vi "DAQ Channels Names.vi"() -> (6 "DAQ channel names (string)":string[](array[string]))   [LabVIEW 2017, in "SignalConverson.lvlib"]
uses:
  SignalConverson.lvlib
  DAQChannelRawData.ctl
panel:
  in  "ChannelNameArray":T1
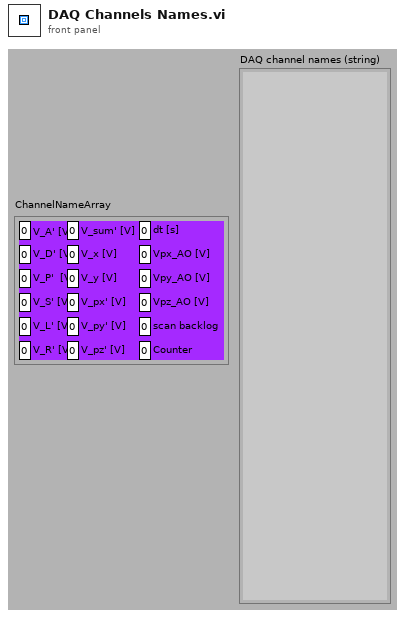
[diagram p1: front panel]
types:
  T1 = typedef "SignalConverson.lvlib/DAQChannelRawData.ctl" = cluster{"V_A' [V]":dbl, "V_D' [V]":dbl, "V_P'  [V]":dbl, "V_S' [V]":dbl, "V_L' [V]":dbl, "V_R' [V]":dbl, "V_sum' [V]":dbl, "V_x [V]":dbl, "V_y [V]":dbl, "V_px' [V]":dbl, "V_py' [V]":dbl, "V_pz' [V]":dbl, "dt [s]":dbl, "Vpx_AO [V]":dbl, "Vpy_AO [V]":dbl, "Vpz_AO [V]":dbl, "scan backlog":u32, "Counter":u32}
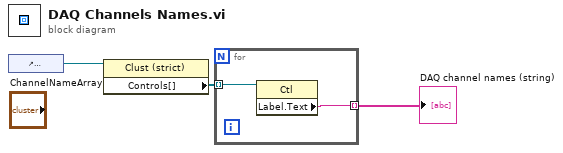
[diagram p0: block diagram]
diagram:
  n1 = control-ref of="ChannelNameArray"() -> (w3:refnum<vi>)
  n2 = property class="Clust (strict)"(reference=w3) -> ("Controls[]"=w1:refnum<vi>[])  [unwired: 1 in, 2 out]
  n3 = for {
    tunnel: [w5] -> w2 mode=indexing
    tunnel: w1 -> [w4] mode=indexing
    n4 = property class="Ctl"(reference=w4) -> ("Label.Text"=w5:string)  [unwired: 1 in, 2 out]
  }
  "DAQ channel names (string)" <- w2
